vi "Untitled 5.vi"(10 "Module Number":dbl, 11 "Controls[]":refnum<vi>[](array[refnum])) -> (1 "Primery key Names":string[](array[string]), 2 "Primery key values":string[](array[string]), 3 "BatchData":string[](array[string]))   [LabVIEW 2015, in "Copy of Untitled Library 1.lvlib"]
uses:
  Copy of Untitled Library 1.lvlib
  Controls/Enum Constant.ctl
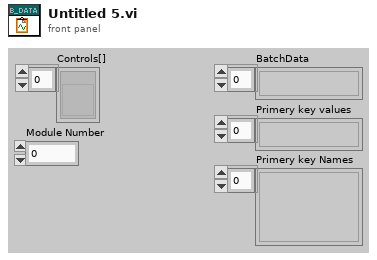
[diagram p1: front panel]
types:
  T1 = typedef "Enum Constant.ctl" = enum16{"Init", "Read", "Write"}
  T2 = typedef "FGV Data.ctl" = T3[]
  T3 = typedef "FGV Cluster Data.ctl" = cluster{"Manual/Automatic":bool, "UI Controllers ":string[], "UI Primery Key ":dbl[], "Caller Queue & MSG":T4, "Module ID":dbl, "DB Reference In":T5, "Products Columns":string[], "Cluster":cluster{"Delete Product":enum8{"Enabled", "Disabled", "Disabled and Grayed Out"}, "Add Product ":enum8{"Enabled", "Disabled", "Disabled and Grayed Out"}, "EDIT BATCH":enum8{"Enabled", "Disabled", "Disabled and Grayed Out"}, "Open Batch ":enum8{"Enabled", "Disabled", "Disabled and Grayed Out"}, "Close Batch":enum8{"Enabled", "Disabled", "Disabled and Grayed Out"}, "Delete Batch":enum8{"Enabled", "Disabled", "Disabled and Grayed Out"}, "Add Batch ":enum8{"Enabled", "Disabled", "Disabled and Grayed Out"}}}
  T4 = typedef "Queue and Caller MSG.ctl" = cluster{"Caller Queue":refnum<queue>, "Caller MSG":string}
  T5 = typedef "NI_Database_API.lvlib/Conn ObjectReference.ctl" = refnum<k1>
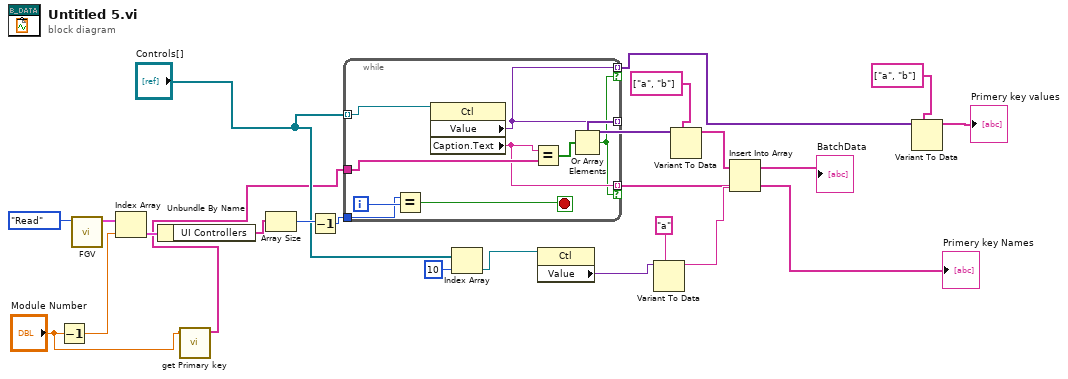
[diagram p0: block diagram]
diagram:
  n1 = Decrement(x="Module Number") -> (x-1=w10:dbl)
  n2 = call "FGV.vi"("Enum"=Enum_Constant."Read") -> ("Read Data"=w20:T2)  [unwired: 9 in, 1 out]
  n3 = Index Array(array=w20, index=w10) -> (element=w19:T3)
  n4 = Unbundle By Name(w19) -> ("UI Controllers"=w7:string[])
  n5 = call "get Primary key.vi"("Module Number"="Module Number") -> ("Primery Key"=w5:string[])  [unwired: 10 in]
  n6 = Array Size(array=w7) -> (size(s)=w23:i32)
  n7 = Decrement(x=w23) -> (x-1=w22:i32)
  n8 = while {
    tunnel: w22 -> [w31]
    tunnel: "Controls[]" -> [w29] mode=indexing
    tunnel: [w27] -> w17 mode=indexing
    tunnel: w5 -> [w28]
    tunnel: [w27] -> w3 mode=indexing if=w24
    tunnel: [w25] -> w1 mode=indexing if=w24
    i -> [w32]
    stop <- w30 stop-if-true
    n9 = Equal?(x=w31, y=w32) -> (x = y?=w30:bool)
    n10 = property class="Ctl"(reference=w29) -> ("Value"=w27:variant, "Caption.Text"=w25:string)  [unwired: 1 in, 2 out]
    n11 = Equal?(x=w25, y=w28) -> (x = y?=w26:bool[])
    n12 = Or Array Elements(Boolean array=w26) -> (logical OR=w24:bool)
  }
  "Primery key Names" <- w1
  n13 = Index Array(array="Controls[]", index=10) -> (element=w15:refnum<vi>)
  n14 = property class="Ctl"(reference=w15) -> ("Value"=w13:variant)  [unwired: 1 in, 2 out]
  n15 = Variant To Data(type="a" ("Caption.Text"), Variant=w13) -> (data=w12:string)  [unwired: 1 in, 1 out]
  n16 = Variant To Data(type=string[] ["a", "b"] ("Array"), Variant=w17) -> (data=w11:string[])  [unwired: 1 in, 1 out]
  n17 = Insert Into Array(array=w11, new element=w12) -> (→"BatchData":string[])  [unwired: 1 in]
  n18 = Variant To Data(type=string[] ["a", "b"] ("Array"), Variant=w3) -> (data=→"Primery key values":string[])  [unwired: 1 in, 1 out]
